vi "Read from XML.vi"() -> ()   [LabVIEW 2019, in "Flattening.lvclass"]
uses:
  Flattening.lvclass
  Flattening.lvclass/Flattening.ctl
panel:
  out "DataValueHere":dbl
  out "Flattening out":refnum<class "Flattening.lvclass">
  in  "Flattening in":refnum<class "Flattening.lvclass">
  out "error out":errorcluster
  in  "error in":errorcluster
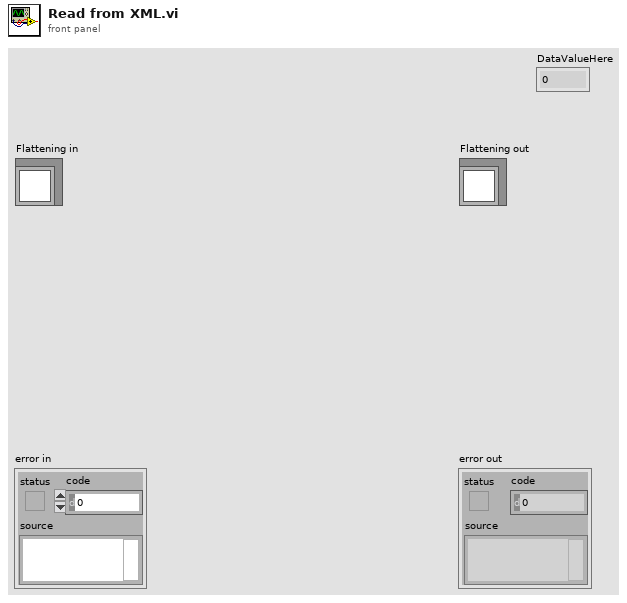
[diagram p1: front panel]
types:
  T1 = enum16{"open", "replace", "create", "open or create", "replace or create", "replace or create with confirmation"}
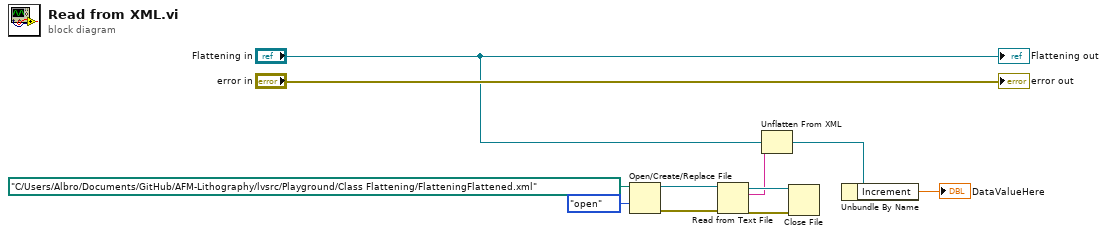
[diagram p0: block diagram]
diagram:
  n1 = Open/Create/Replace File(file path (use dialog)=path "C:/Users/Albro/Documents/GitHub/AFM-Lithography/lvsrc/Playground/Class Flattening/FlatteningFlattened.xml", operation (0:open)=T1."open") -> (refnum out=w11:refnum<file>, error out=w10:errorcluster)  [unwired: 4 in, 1 out]
  n2 = Read from Text File(file (use dialog)=w11, error in=w10) -> (refnum out=w9:refnum<file>, text=w4:string, error out=w8:errorcluster)  [unwired: 2 in, 1 out]
  n3 = Unflatten From XML(xml string=w4, type="Flattening in") -> (value=w2:refnum<class "Flattening.lvclass">)  [unwired: 1 in, 1 out]
  n4 = Close File(refnum=w9, error in=w8) -> ()  [unwired: 2 out]
  n5 = Unbundle By Name(w2) -> ("Increment"=→"DataValueHere":dbl)
  "error out" <- "error in"
  "Flattening out" <- "Flattening in"
